vi "Get Identifier.vi"(8 "error in":errorcluster, 11 "PCAN-USB Read-Write Raw CAN Frame Strategy in":refnum<class "PCAN Base Strategy.lvclass">) -> (0 "error out":errorcluster, 2 "Instrument Identifier":string, 3 "PCAN-USB Read-Write Raw CAN Frame Strategy out":refnum<class "PCAN Base Strategy.lvclass">)   [LabVIEW 2024, in "PCAN Base Strategy.lvclass"]
uses:
  PCAN Base Strategy.lvclass
  PCAN Base Strategy.lvclass/PCAN Base Strategy.ctl
  Source/Interfaces/IConfiguration/IConfiguration.lvclass
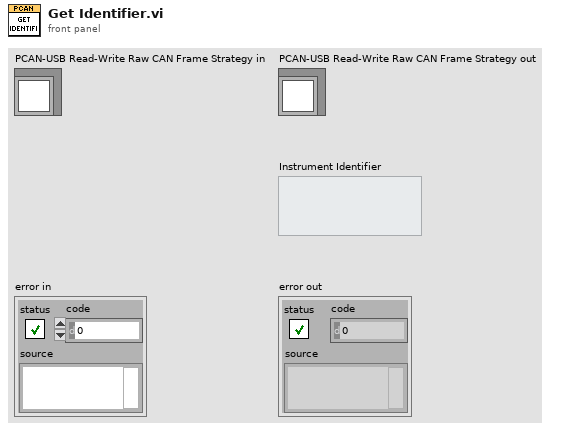
[diagram p1: front panel]
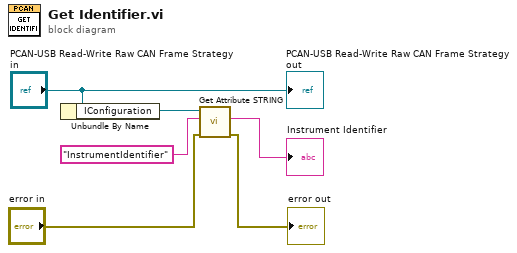
[diagram p0: block diagram]
diagram:
  n1 = Unbundle By Name("PCAN-USB Read-Write Raw CAN Frame Strategy in") -> ("IConfiguration"=w5:refnum<class "IConfiguration.lvclass">)
  n2 = call-dynamic "Get Attribute STRING.vi"("error in"="error in", "Attribute"="InstrumentIdentifier", "IConfiguration in"=w5) -> ("error out"=→"error out":errorcluster, "Value"=→"Instrument Identifier":string)  [unwired: 6 in, 1 out]
  "PCAN-USB Read-Write Raw CAN Frame Strategy out" <- "PCAN-USB Read-Write Raw CAN Frame Strategy in"
